vi "Main.vi"() -> ()   [LabVIEW 2013]
uses:
  PCTx Files/PCTx/PCTx.lvlib
  <vilib>/Utility/inputDevices.llb/joystickAcquire.vi
  TypeDefs/Throttle.ctl
  TypeDefs/Wheel Buttons.ctl
  TypeDefs/Wheel Axes.ctl
  TypeDefs/Steering.ctl
panel:
  in  "Steering Cluster":T1={"Neutral Signal"=642.8571428571429, "Bottom Deadzone"=707.070707070707, "Neutral Deadzone"=0.0, "Top Cutout"=971.4285714285714, "Bottom Cutout"=89.79591836734694, "Top Deadzone"=64627.90909090909, "Throttle Curve Type"=enum."Linear"} {"Top Deadzone" scale=32768.0..65537.0; "Bottom Cutout" scale=0.0..512.0; "Top Cutout" scale=800.0..1024.0; "Neutral Deadzone" scale=0.0..10000.0; "Bottom Deadzone" scale=1.0..32767.0; "Neutral Signal" scale=420.0..700.0}
  out "button info":T2
  out "Raw Wheel Inputs":T3
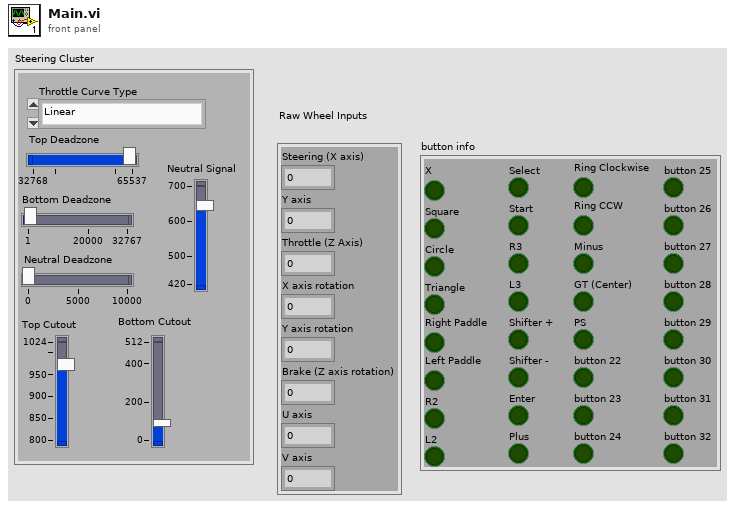
[diagram p1: front panel]
types:
  T1 = typedef "Steering.ctl" = cluster{"Neutral Signal":dbl, "Bottom Deadzone":dbl, "Neutral Deadzone":dbl, "Top Cutout":dbl, "Bottom Cutout":dbl, "Top Deadzone":dbl, "Throttle Curve Type":enum16{"Linear", "Linear, No Deadzone", "Logarithmic", "Exponental"}}
  T2 = typedef "Wheel Buttons.ctl" = cluster{"X":bool, "Square":bool, "Circle":bool, "Triangle":bool, "Right Paddle":bool, "Left Paddle":bool, "R2":bool, "L2":bool, "Select":bool, "Start":bool, "R3":bool, "L3":bool, "Shifter +":bool, "Shifter -":bool, "Enter":bool, "Plus":bool, "Ring Clockwise":bool, "Ring CCW":bool, "Minus":bool, "GT (Center)":bool, "PS":bool, "button 22":bool, "button 23":bool, "button 24":bool, "button 25":bool, "button 26":bool, "button 27":bool, "button 28":bool, "button 29":bool, "button 30":bool, "button 31":bool, "button 32":bool}
  T3 = typedef "Wheel Axes.ctl" = cluster{"Steering (X axis)":i32, "Y axis":i32, "Throttle (Z Axis)":i32, "X axis rotation":i32, "Y axis rotation":i32, "Brake (Z axis rotation)":i32, "U axis":i32, "V axis":i32}
  T4 = enum16{"Set Axes", "Read Axes", "Set Buttons", "Read Buttons", "Get Scaled Throttle", "Get Scaled Steering", "Get Scaled Brake"}
  T5 = typedef "Throttle.ctl" = cluster{"Neutral Signal":dbl, "Bottom Deadzone":dbl, "Neutral Deadzone":dbl, "Top Cutout":dbl, "Bottom Cutout":dbl, "Top Deadzone":dbl, "Throttle Curve Type":enum16{"Linear", "Linear, No Deadzone", "Logarithmic", "Exponental"}}
  T6 = cluster{"X axis":i32, "Y axis":i32, "Z axis":i32, "X axis rotation":i32, "Y axis rotation":i32, "Z axis rotation":i32, "U axis":i32, "V axis":i32}
  T7 = cluster{"button 1":bool, "button 2":bool, "button 3":bool, "button 4":bool, "button 5":bool, "button 6":bool, "button 7":bool, "button 8":bool, "button 9":bool, "button 10":bool, "button 11":bool, "button 12":bool, "button 13":bool, "button 14":bool, "button 15":bool, "button 16":bool, "button 17":bool, "button 18":bool, "button 19":bool, "button 20":bool, "button 21":bool, "button 22":bool, "button 23":bool, "button 24":bool, "button 25":bool, "button 26":bool, "button 27":bool, "button 28":bool, "button 29":bool, "button 30":bool, "button 31":bool, "button 32":bool}
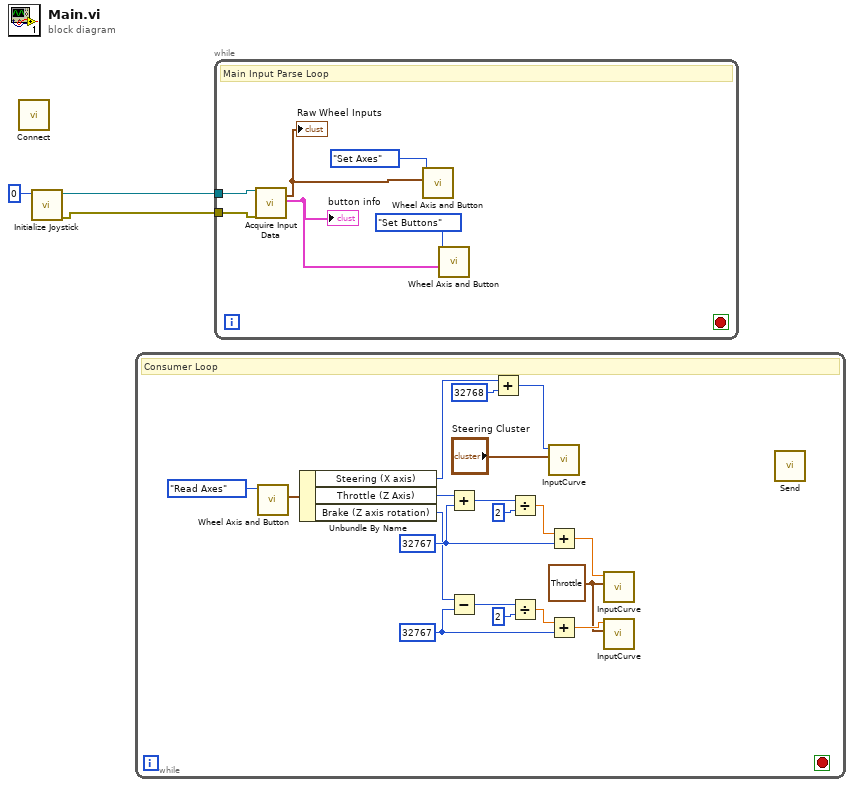
[diagram p0: block diagram]
diagram:
  n1 = call "Connect.vi"() -> ()  [unwired: 10 in, 2 out]
  n2 = call <vilib>:"Initialize Joystick.vi"("device index"=0) -> ("error out"=w1:errorcluster, "device ID"=w2:refnum<k1>)  [unwired: 9 in]
  n3 = while {
    stop <- _ stop-if-true
    w6 = T5 {"Neutral Signal"=512.0, "Bottom Deadzone"=707.070707070707, "Neutral Deadzone"=0.0, "Top Cutout"=971.4285714285714, "Bottom Cutout"=89.79591836734694, "Top Deadzone"=64627.90909090909, "Throttle Curve Type"=enum."Linear"} ("Throttle Cluster")
    w13 = 32767 ("x")
    w14 = 32767 ("x")
    # "Consumer Loop"
    n4 = call "Wheel Axis and Button.vi"("Action"=T4."Read Axes") -> ("Raw Wheel Axes"=w18:T3)  [unwired: 9 in, 1 out]
    n5 = Unbundle By Name(w18) -> ("Steering (X axis)"=w16:i32, "Throttle (Z Axis)"=w15:i32, "Brake (Z axis rotation)"=w10:i32)
    n6 = Add(x=w15, y=w14) -> (x+y=w20:i32)
    n7 = Subtract(x=w10, y=w13) -> (x-y=w9:i32)
    n8 = Add(x=w16, y=32768 ("x")) -> (x+y=w5:i32)
    n9 = Divide(x=w20, y=2) -> (x/y=w22:dbl)
    n10 = Divide(x=w9, y=2) -> (x/y=w11:dbl)
    n11 = call "InputCurve.vi"("Throttle Cluster"="Steering Cluster", "Input"=w5) -> ()  [unwired: 8 in, 2 out]
    n12 = Add(x=w22, y=w14) -> (x+y=w8:dbl)
    n13 = Add(x=w11, y=w13) -> (x+y=w7:dbl)
    n14 = call "InputCurve.vi"("Throttle Cluster"=w6, "Input"=w8) -> ()  [unwired: 8 in, 2 out]
    n15 = call "InputCurve.vi"("Throttle Cluster"=w6, "Input"=w7) -> ()  [unwired: 8 in, 2 out]
    n16 = call "Send.vi"() -> ()  [unwired: 26 in, 2 out]
  }
  n17 = while {
    tunnel: w2 -> [w28]
    tunnel: w1 -> [w27]
    stop <- _ stop-if-true
    # "Main Input Parse Loop"
    n18 = call-poly <vilib>:"Acquire Input Data.vi"("device ID"=w28, "error in (no error)"=w27) -> ("axis info"=w25:T6, "button info"=w24:T7)  [unwired: 13 in, 3 out]
    "Raw Wheel Inputs" <- w25
    "button info" <- w24
    n19 = call "Wheel Axis and Button.vi"("Raw Wheel Axes"=w25, "Action"=T4."Set Axes") -> ()  [unwired: 8 in, 2 out]
    n20 = call "Wheel Axis and Button.vi"("Wheel Button Input"=w24, "Action"=T4."Set Buttons") -> ()  [unwired: 8 in, 2 out]
  }
